vi "Create Sysdef and Add New Custom Device.vi"() -> ()   [LabVIEW 2010]
uses:
  Read RefMem PtByPt System Definition API.lvlibp/API/Channel Config.ctl
  Read RefMem PtByPt System Definition API.lvlibp/Custom Device/Controls/Data Channel Type.ctl
  NationalInstruments.VeriStand.SystemDefinitionAPI
  Read RefMem PtByPt System Definition API.lvlibp
  Read RefMem PtByPt System Definition API.lvlibp/Custom Device/RefMem PtByPt Custom Device.lvlib
panel:
  in  "Decimation":i32=1
  in  "CPU Assignment":i32=-2
  in  "VISA Name":string="RM"
  in  "Data Folder to Add":string="MyFolder"
  in  "Data Channel Config":T1[](array[typedef])=[{"Units"="blah", "Default Value"=0.0, "Address"=0, "Description"="", "Type"=enum."Read"}, {"Units"="blah", "Default Value"=1.0, "Address"=8, "Description"="", "Type"=enum."Read"}] {"Address" format="%.0x"}
  in  "Data Channels to Add to Folder":string[](array[string])=["MyChan1", "MyChan2"]
  in  "Device Name":string="My RefMem Reader"
  in  "Sysdef File to create":path
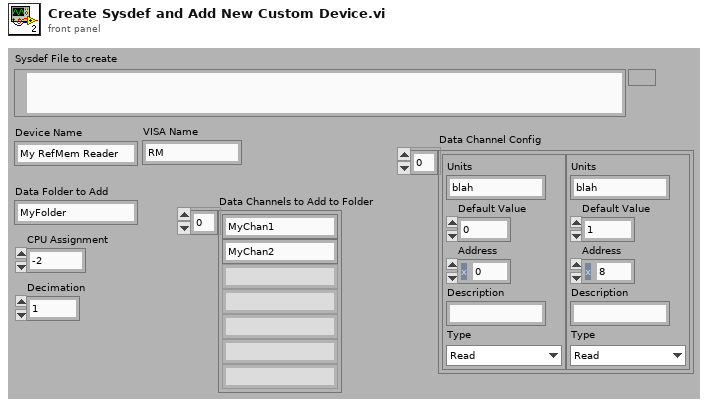
[diagram p1: front panel]
types:
  T1 = typedef "Read RefMem PtByPt System Definition API.lvlibp/Channel Config.ctl" = cluster{"Units":string, "Default Value":dbl, "Address":u32, "Description":string, "Type":T2}
  T2 = typedef "Read RefMem PtByPt System Definition API.lvlibp/RefMem PtByPt Custom Device.lvlib/Data Channel Type.ctl" = enum16{"Read", "Write"}
  T3 = typedef "SysDefRefs.ctl" = cluster{"SysDef Ref":refnum<k24>, "Root Node":refnum<k24>, "Targets Section":refnum<k24>, "Target List":refnum<k24>[], "CD Section":refnum<k24>, "CustomDeviceList":refnum<k24>[]}
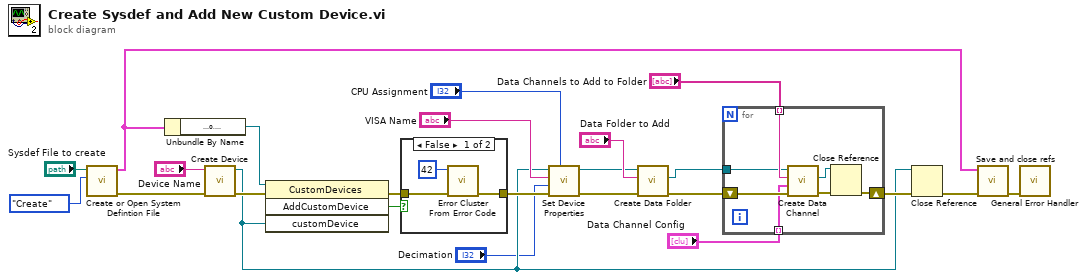
[diagram p0: block diagram]
diagram:
  n1 = call "Create or Open System Defintion File.vi"("File Action"=enum16{"Open", "Create"}."Create", "Sysdef File"="Sysdef File to create") -> ("error out"=w16:errorcluster, "SysDef Refs"=w20:T3)  [unwired: 8 in]
  n2 = Unbundle By Name(w20) -> ("CD Section"=w19:refnum<k24>)
  n3 = call "Create Device.vi"("error in (no error)"=w16, "Name"="Device Name") -> ("error out"=w6:errorcluster, "Custom Device"=w3:refnum<k24>)  [unwired: 8 in]
  n4 = invoke class="CustomDevices" method="AddCustomDevice"(reference=w19, error in=w6, "customDevice"=w3) -> (error out=w22:errorcluster, "AddCustomDevice"=w21:bool)  [unwired: 1 in, 2 out]
  n5 = case shown="False" w21 {
    tunnel: [w26 w28] -> w5
    tunnel: w22 -> [w25 w28]
    frame False {
      n6 = call <vilib>:"Error Cluster From Error Code.vi"("error in (no error)"=w25, "error code (0)"=42) -> ("error out"=w26:errorcluster)  [unwired: 7 in]
    }
    frame True {
    }
  }
  n7 = call "Set Device Properties.vi"("CPU Assignment (-2)"="CPU Assignment", "error in (no error)"=w5, "Decimation (1)"="Decimation", "VISA Name"="VISA Name", "Custom Device"=w3) -> ("error out"=w9:errorcluster, "Custom Device Duplicate"=w10:refnum<k24>)  [unwired: 5 in]
  n8 = call "Create Data Folder.vi"("error in (no error)"=w9, "Name"="Data Folder to Add", "Parent Section"=w10) -> ("error out"=w14:errorcluster, "New Section"=w13:refnum<k24>)  [unwired: 5 in, 2 out]
  n9 = for {
    shift-right: [w31] -> w4
    shift-left: w14 -> [w35]
    tunnel: "Data Channels to Add to Folder" -> [w34] mode=indexing
    tunnel: w13 -> [w33]
    tunnel: "Data Channel Config" -> [w32] mode=indexing
    n10 = call "Create Data Channel.vi"("error in (no error)"=w35, "Channel"=w32, "Name"=w34, "Parent Section"=w33) -> ("error out"=w30:errorcluster, "New Data Channel"=w29:refnum<k24>)  [unwired: 3 in, 3 out]
    n11 = Close Reference(reference=w29, error in (no error)=w30) -> (error out=w31:errorcluster)
  }
  n12 = Close Reference(reference=w3, error in (no error)=w4) -> (error out=w7:errorcluster)
  n13 = call "Save and close refs.vi"("error in (no error)"=w7, "SysDef Refs in"=w20) -> ("error out"=w23:errorcluster)  [unwired: 9 in]
  n14 = call <vilib>:"General Error Handler.vi"("error in (no error)"=w23) -> ()  [unwired: 10 in, 5 out]
